vi "PlotLangevinCore.vi"(4 "PointsToPlot":i32=84, 7 "Peak mT":dbl=11.901571409662573, 8 "Normalize to mass?":bool=TRUE, 9 "MassKg":dbl=5e-09 format="%#.2p", 10 "BMon":dbl[](array[numeric])=array[12600 elements], 11 "Rx":dbl[](array[numeric])=array[12600 elements]) -> (0 "BMon_Int_mT":dbl[](array[numeric])=[-11.752058348361746, -11.816218197086325, -11.814368466853411, -11.746509159619366, -11.611885882176448, -11.411253031562175, -11.147250992471712, -10.821011359254825, -10.433665726104367, -9.987854477204506, -9.485463601516331, -8.92951068033226, -8.323390492256122, -7.670120618171406, -6.973850231220703, -6.239482899272534, -5.470413400115998, -4.6696593139119855, -3.8425014054640827, -2.993088847057799, -2.1267024032090402, -1.249000035799517, -0.3645081142752374, 0.5226241893990321, 1.4074933083723242, 2.28444128087955, 3.1489417374608855, 3.9968455060516033, 4.822871822118466, 5.620985526082497, 6.387791840440792, 7.118764395123147, 7.809754017378031, 8.45774312667623, 9.058959747361609, 9.610386298551257, 10.107873606633136, 10.549535682863551, 10.933109340746633, 11.25482260353677, 11.513543876978385, 11.70814156669706, 11.837861275789038, 11.901571409662573, 11.898517571234919, 11.829831351321603, 11.695889945573102, 11.496693352058971, 11.233373161726012, 10.906683767941319, 10.51888835478979, 10.072627304142564, 9.570163800447903, 9.014892621357763, 8.40983134708351, 7.757620360338971, 7.062031637171542, 6.326837153832879, 5.555808886822503, 4.753850406017957, 3.92586528152873, 3.0767570836509, 2.2106749873491545, 1.3321453654460547, 0.44607178859401186, -0.4418877769992446, -1.327206958353787, -2.204982184765175, -3.069555490089271, -3.917532094741724, -4.743631230552419, -5.542572129500532, -6.310205616978582, -7.042382518554533, -7.735330857741325, -8.38527865825331, -8.987699548674373, -9.539198750904397, -10.037513080164219, -10.480002154139003, -10.863271195444261, -11.185057019830644, -11.444982431454598, -11.641161443988233], 1 "Rx_M_t_Out":dbl[](array[numeric])=[-94.99013348437892, -96.28276872749046, -97.23009881656009, -97.86284033654283, -98.32465355727314, -98.5386948514044, -98.79705481345721, -98.87004982206153, -98.84756646146671, -98.77569917375844, -98.26497805054365, -97.7095162602339, -96.83899202839694, -96.08495135140485, -94.99102676674816, -93.98470760182397, -92.45126761302751, -90.552553370214, -88.18762318621485, -85.33744237035638, -81.64474117324269, -76.73750964557067, -69.67504193754885, -59.86681915549513, -46.71377648212639, -31.76346316111322, -16.704091001308953, -2.33582475921248, 11.106008516197418, 23.651711703953158, 35.165588045060744, 45.762792483863436, 55.057889459257595, 63.19858779341371, 70.04201228419701, 75.70980856156083, 80.20395831191821, 83.9166637616591, 86.9834948356949, 89.71419618141137, 91.86049527411762, 93.62158730018476, 94.95437964378733, 96.08982618873921, 96.89804450658906, 97.55845873875946, 98.14180556951518, 98.60688887332236, 98.90088908414768, 98.95907743361799, 98.72194363291179, 98.43657855234228, 97.96895772499005, 97.57977866098764, 96.89608792349443, 96.1020578975974, 94.97527082633499, 93.6524386624182, 92.09715969163996, 90.2023640742574, 88.14988047969908, 85.33526751441805, 81.86791902743036, 76.82377980787773, 69.74238884614049, 59.83167453612357, 46.86571619899478, 32.06238679736975, 17.174882179179413, 2.7997285686522475, -10.766907232320722, -23.454369451760687, -35.23721571036733, -45.69607883367942, -54.94663378956453, -62.86616960491522, -69.75074749980371, -75.49197094927564, -80.24211534445327, -84.1236008376034, -87.22238080615581, -89.81883140016181, -91.81122878308248, -93.59828995170739], 2 "BMon Int":dbl[](array[numeric]), 3 "Rx_M_t":dbl[](array[numeric]))   [LabVIEW 2021]
uses:
  MPS_global_variables.vi
panel:
  out "t2":dbl
  out "Real":dbl
  out "size(s)":i32[](array[numeric])=[1, 12600]
  out "Waveform Graph":dbl[](graph)=[-11.752058348361746, -11.816218197086325, -11.814368466853411, -11.746509159619366, -11.611885882176448, -11.411253031562175, -11.147250992471712, -10.821011359254825, -10.433665726104367, -9.987854477204506, -9.485463601516331, -8.92951068033226, -8.323390492256122, -7.670120618171406, -6.973850231220703, -6.239482899272534, -5.470413400115998, -4.6696593139119855, -3.8425014054640827, -2.993088847057799, -2.1267024032090402, -1.249000035799517, -0.3645081142752374, 0.5226241893990321, 1.4074933083723242, 2.28444128087955, 3.1489417374608855, 3.9968455060516033, 4.822871822118466, 5.620985526082497, 6.387791840440792, 7.118764395123147, 7.809754017378031, 8.45774312667623, 9.058959747361609, 9.610386298551257, 10.107873606633136, 10.549535682863551, 10.933109340746633, 11.25482260353677, 11.513543876978385, 11.70814156669706, 11.837861275789038, 11.901571409662573, 11.898517571234919, 11.829831351321603, 11.695889945573102, 11.496693352058971, 11.233373161726012, 10.906683767941319, 10.51888835478979, 10.072627304142564, 9.570163800447903, 9.014892621357763, 8.40983134708351, 7.757620360338971, 7.062031637171542, 6.326837153832879, 5.555808886822503, 4.753850406017957, 3.92586528152873, 3.0767570836509, 2.2106749873491545, 1.3321453654460547, 0.44607178859401186, -0.4418877769992446, -1.327206958353787, -2.204982184765175, -3.069555490089271, -3.917532094741724, -4.743631230552419, -5.542572129500532, -6.310205616978582, -7.042382518554533, -7.735330857741325, -8.38527865825331, -8.987699548674373, -9.539198750904397, -10.037513080164219, -10.480002154139003, -10.863271195444261, -11.185057019830644, -11.444982431454598, -11.641161443988233]
  out "XY Graph":cluster{"Y":dbl[], "Y":dbl[]}[](graph)=[{"Y"=[-11.752058348361746, -11.816218197086325, -11.814368466853411, -11.746509159619366, -11.611885882176448, -11.411253031562175, -11.147250992471712, -10.821011359254825, -10.433665726104367, -9.987854477204506, -9.485463601516331, -8.92951068033226, -8.323390492256122, -7.670120618171406, -6.973850231220703, -6.239482899272534, -5.470413400115998, -4.6696593139119855, -3.8425014054640827, -2.993088847057799, -2.1267024032090402, -1.249000035799517, -0.3645081142752374, 0.5226241893990321, 1.4074933083723242, 2.28444128087955, 3.1489417374608855, 3.9968455060516033, 4.822871822118466, 5.620985526082497, 6.387791840440792, 7.118764395123147, 7.809754017378031, 8.45774312667623, 9.058959747361609, 9.610386298551257, 10.107873606633136, 10.549535682863551, 10.933109340746633, 11.25482260353677, 11.513543876978385, 11.70814156669706, 11.837861275789038, 11.901571409662573, 11.898517571234919, 11.829831351321603, 11.695889945573102, 11.496693352058971, 11.233373161726012, 10.906683767941319, 10.51888835478979, 10.072627304142564, 9.570163800447903, 9.014892621357763, 8.40983134708351, 7.757620360338971, 7.062031637171542, 6.326837153832879, 5.555808886822503, 4.753850406017957, 3.92586528152873, 3.0767570836509, 2.2106749873491545, 1.3321453654460547, 0.44607178859401186, -0.4418877769992446, -1.327206958353787, -2.204982184765175, -3.069555490089271, -3.917532094741724, -4.743631230552419, -5.542572129500532, -6.310205616978582, -7.042382518554533, -7.735330857741325, -8.38527865825331, -8.987699548674373, -9.539198750904397, -10.037513080164219, -10.480002154139003, -10.863271195444261, -11.185057019830644, -11.444982431454598, -11.641161443988233], "Y"=[-94.99013348437892, -96.28276872749046, -97.23009881656009, -97.86284033654283, -98.32465355727314, -98.5386948514044, -98.79705481345721, -98.87004982206153, -98.84756646146671, -98.77569917375844, -98.26497805054365, -97.7095162602339, -96.83899202839694, -96.08495135140485, -94.99102676674816, -93.98470760182397, -92.45126761302751, -90.552553370214, -88.18762318621485, -85.33744237035638, -81.64474117324269, -76.73750964557067, -69.67504193754885, -59.86681915549513, -46.71377648212639, -31.76346316111322, -16.704091001308953, -2.33582475921248, 11.106008516197418, 23.651711703953158, 35.165588045060744, 45.762792483863436, 55.057889459257595, 63.19858779341371, 70.04201228419701, 75.70980856156083, 80.20395831191821, 83.9166637616591, 86.9834948356949, 89.71419618141137, 91.86049527411762, 93.62158730018476, 94.95437964378733, 96.08982618873921, 96.89804450658906, 97.55845873875946, 98.14180556951518, 98.60688887332236, 98.90088908414768, 98.95907743361799, 98.72194363291179, 98.43657855234228, 97.96895772499005, 97.57977866098764, 96.89608792349443, 96.1020578975974, 94.97527082633499, 93.6524386624182, 92.09715969163996, 90.2023640742574, 88.14988047969908, 85.33526751441805, 81.86791902743036, 76.82377980787773, 69.74238884614049, 59.83167453612357, 46.86571619899478, 32.06238679736975, 17.174882179179413, 2.7997285686522475, -10.766907232320722, -23.454369451760687, -35.23721571036733, -45.69607883367942, -54.94663378956453, -62.86616960491522, -69.75074749980371, -75.49197094927564, -80.24211534445327, -84.1236008376034, -87.22238080615581, -89.81883140016181, -91.81122878308248, -93.59828995170739]}]
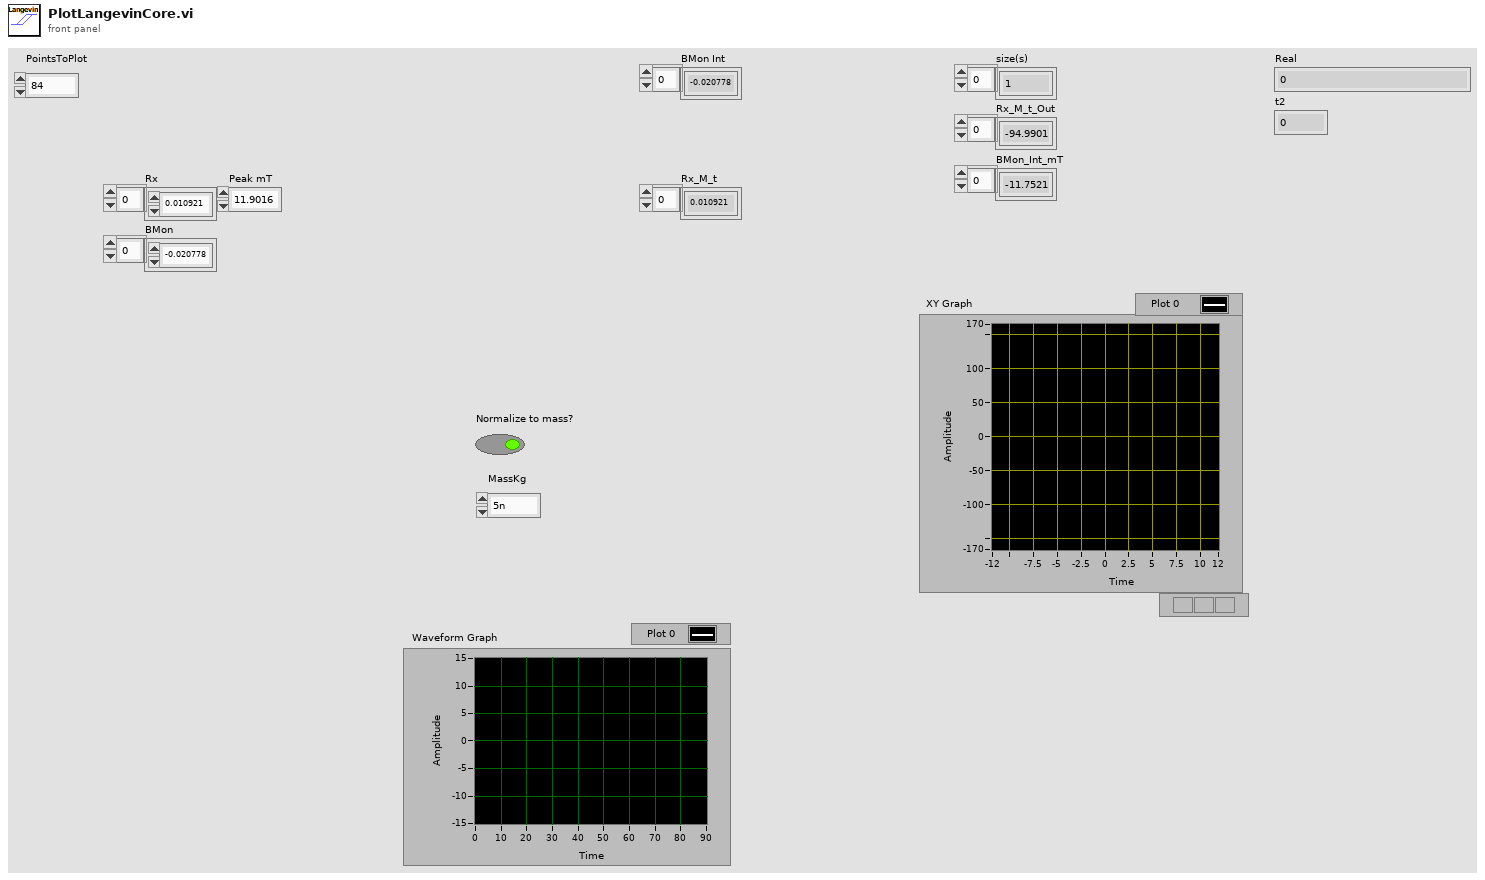
[diagram p1: front panel]
types:
  T1 = cluster{"sample rate":dbl, "Tx freq":dbl, "Tx amp":dbl, "Tx cycles\nSpectroscopy":dbl, "Bias amp":dbl, "Bias freq":dbl, "Receive range":dbl, "Bias Periods\nMagnetometry":dbl, "Tx Freq Division Factor":dbl, "Drive Periods per Bias":dbl, "TX harmonics":dbl[]}
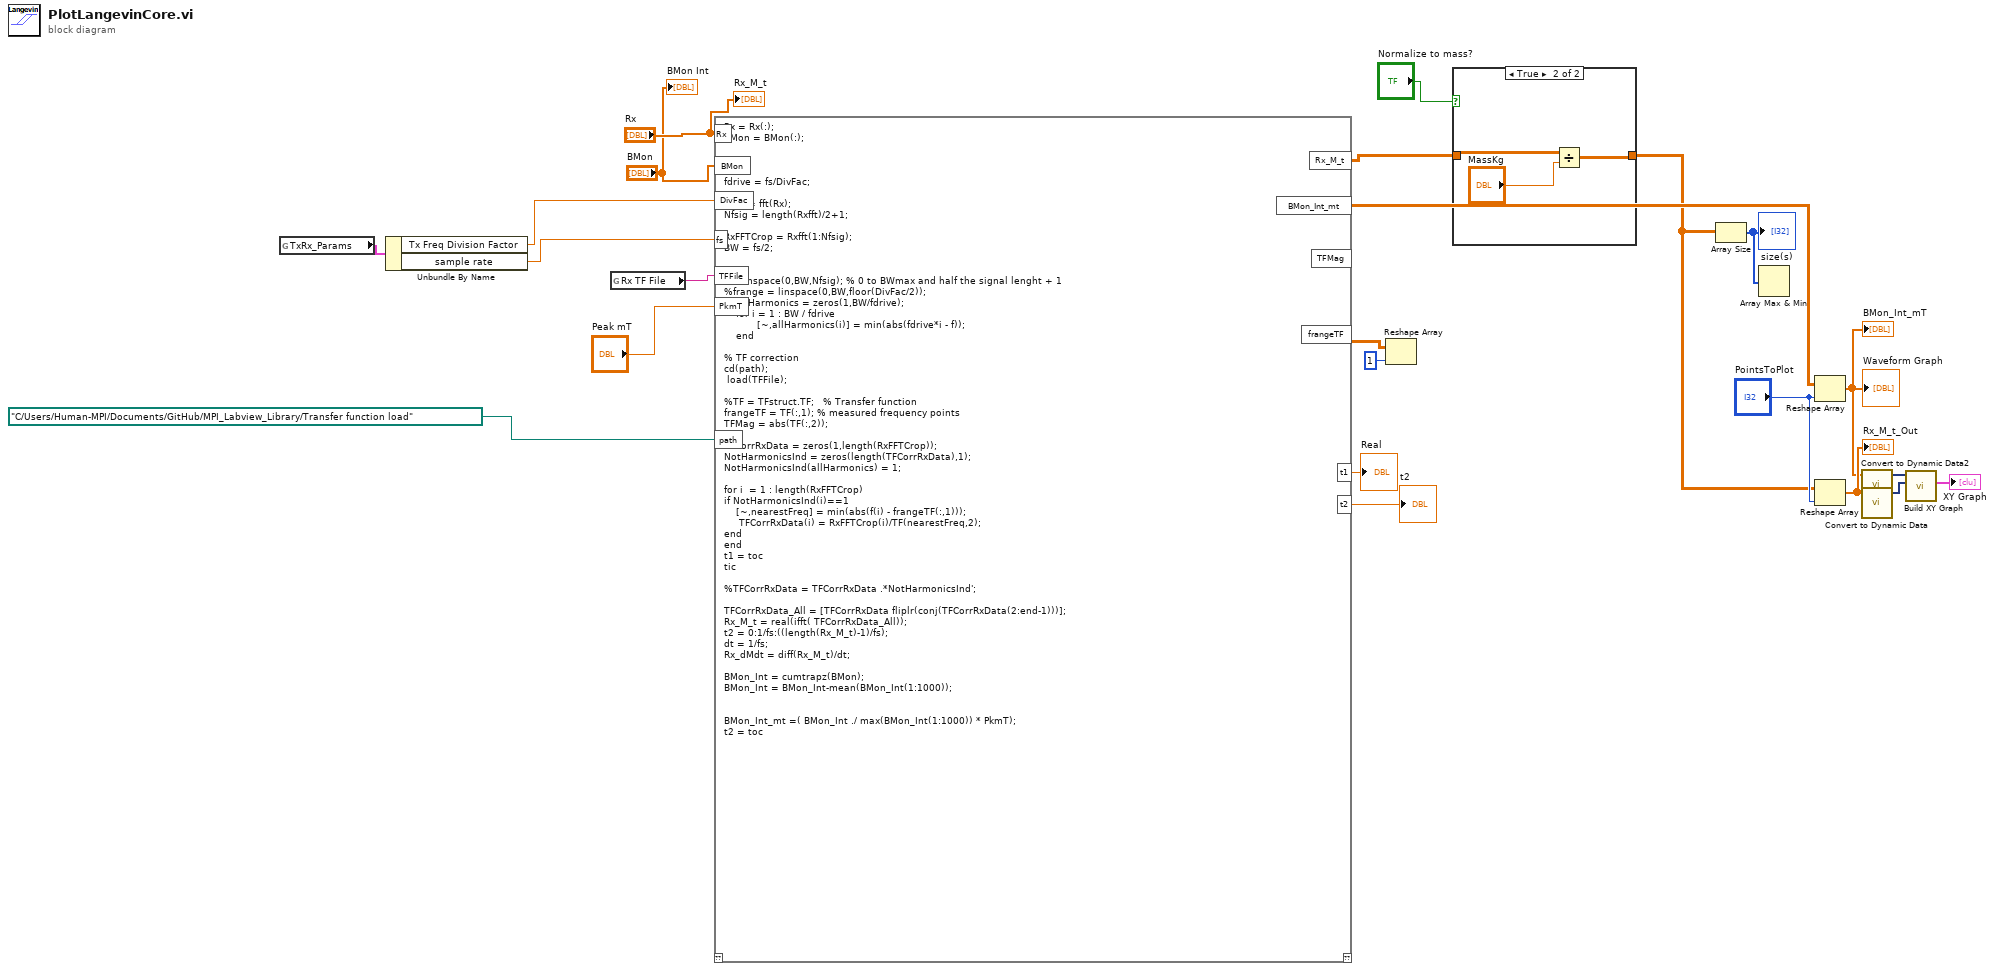
[diagram p0: block diagram]
diagram:
  n1 = global read "MPS_global_variables.vi" "TxRx_Params"() -> (w23:T1)
  n2 = Unbundle By Name(w23) -> ("Tx Freq Division Factor"=w22:dbl, "sample rate"=w21:dbl)
  n3 = global read "MPS_global_variables.vi" "Rx TF File"() -> (w20:string)
  n4 = script code="Rx = Rx(:);\nBMon = BMon(:);\n\n\n\nfdrive = fs/DivFac;\n\nRxfft = fft(Rx);\nNfsig = length(Rxfft)/2+1;\n\nRxFFTCrop = Rxfft(1:Nfsig);\nBW = fs/2;\n \n\nf = linspace(0,BW,Nfsig); % 0 to BWmax and half the signal lenght + 1\n%frange = linspace(0,BW,floor(DivFac/2));\n    allHarmonics = zeros(1,BW/fdrive);\n    for i = 1 : BW / fdrive\n           [~,allHarmonics(i)] = min(abs(fdrive*i - f));\n    end\n\n% TF correction\ncd(path);\n load(TFFile);\n\n%TF = TFstruct.TF;   % Transfer function\nfrangeTF = TF(:,1); % measured frequency points\nTFMag = abs(TF(:,2));\ntic\nTFCorrRxData = zeros(1,length(RxFFTCrop));\nNotHarmonicsInd = zeros(length(TFCorrRxData),1);\nNotHarmonicsInd(allHarmonics) = 1;\n\nfor i  = 1 : length(RxFFTCrop)\nif NotHarmonicsInd(i)==1\n    [~,nearestFreq] = min(abs(f(i) - frangeTF(:,1)));\n     TFCorrRxData(i) = RxFFTCrop(i)/TF(nearestFreq,2);\nend\nend\nt1 = toc\ntic\n\n%TFCorrRxData = TFCorrRxData .*NotHarmonicsInd';\n\nTFCorrRxData_All = [TFCorrRxData fliplr(conj(TFCorrRxData(2:end-1)))];\nRx_M_t = real(ifft( TFCorrRxData_All));\nt2 = 0:1/fs:((length(Rx_M_t)-1)/fs);\ndt = 1/fs;\nRx_dMdt = diff(Rx_M_t)/dt;\n\nBMon_Int = cumtrapz(BMon);\nBMon_Int = BMon_Int-mean(BMon_Int(1:1000));\n\n\nBMon_Int_mt =( BMon_Int ./ max(BMon_Int(1:1000)) * PkmT);\nt2 = toc"("Rx"="Rx", "DivFac"=w22, "fs"=w21, "BMon"="BMon", "TFFile"=w20, "PkmT"="Peak mT", "path"=path "C:/Users/Human-MPI/Documents/GitHub/MPI_Labview_Library/Transfer function load" ("path for measured TF mat file")) -> ("Rx_M_t"=w3:dbl[][], "BMon_Int_mt"=w8:dbl[][], "frangeTF"=w12:dbl[][], "t1"=→"Real":dbl, "t2"=→"t2":dbl)  [unwired: 1 in, 2 out]
  n5 = Reshape Array(w12, 1 ("dimension size")) -> ()  [unwired: 1 out]
  n6 = case shown="True" "Normalize to mass?" {
    tunnel: [w24 w27] -> w4
    tunnel: w3 -> [w24 w25]
    frame False {
    }
    frame True {
      n7 = Divide(x=w25, y="MassKg") -> (x/y=w27:dbl[][])
    }
  }
  n8 = Array Size(array=w4) -> (size(s)=w10:i32[])
  "size(s)" <- w10
  n9 = Array Max & Min(array=w10) -> ()  [unwired: 4 out]
  n10 = Reshape Array(w8, "PointsToPlot") -> (w6:dbl[])
  "Waveform Graph" <- w6
  "BMon_Int_mT" <- w6
  n11 = Reshape Array(w4, "PointsToPlot") -> (w9:dbl[])
  "Rx_M_t_Out" <- w9
  n12 = call "Convert to Dynamic Data2"("Array"=w6) -> ("Dynamic Data Type"=w14:dynamicdata)  [unwired: 3 in]
  n13 = call "Convert to Dynamic Data"("Array"=w9) -> ("Dynamic Data Type"=w15:dynamicdata)  [unwired: 3 in]
  n14 = call "Build XY Graph"("Y Input"=w15, "X Input"=w14) -> ("XY Graph"=→"XY Graph":cluster{"X":dbl[], "Y":dbl[]}[])  [unwired: 8 in, 1 out]
  "Rx_M_t" <- "Rx"
  "BMon Int" <- "BMon"
